vi "DCS_1_(Upgrade).vi"(3 "error in":errorcluster) -> (10 "error out":errorcluster)   [LabVIEW 2013]
uses:
  <vilib>/Utility/miscctls.llb/LVPointTypeDef.ctl
  <userlib>/Accelerator/User Interface/Controls/Role ID.ctl
  <userlib>/Accelerator/User Interface/Controls/dcs_spot.ctl
  <vilib>/gmath/NumericalOptimization/Nonlinear Curve Fit LM.vi
  <userlib>/Accelerator/User Interface/Controls/dcs points.ctl
  <vilib>/gmath/NI_Gmath.lvlib
panel:
  in  "Waveform Path":path=path "C:/Users/Chris/Desktop/DCS(Upgrade)/Waveforms"
  in  "Nornamiled":path=path "C:/Users/Chris/Desktop/DCS(Upgrade)/dcs_data/dcs_normalized.csv"
  in  "XY and Max":path=path "C:/Users/Chris/Desktop/DCS(Upgrade)/dcs_points/dcs_points.csv"
  in  "Points to Check Noise":i32=2000
  in  "Color bar Control":cluster{dbl, u32}[](array[cluster])
  in  "stop":bool
  in  "Tab Control":T1(tab)
  out "Intensity Graph":dbl[][](graph)
  in  "Spot Save Folder":path=path "C:/Users/Chris/Desktop/DCS(Upgrade)/dcs_data"
  in  "Save Spot Image":bool
  in  "Clear Spot/Track":bool
  in  "Particle Limit":i64=500 min=0 step=10
  out "Laser spot\nMove (mm)":dbl[](array[numeric])=[nan, nan] format="%#.3g"
  out "Avg. Freq. (Hz)":dbl
  in  "Orange Cursor Position":dbl[](array[numeric])=[0.0, 0.0] min=-12.0 max=12.0 step=0.1 format="%.3g"
  out "Spot Widths":dbl[](array[numeric]) format="%.6g"
  out "Countdown to\nnext track point":i32=1
  out "XY Graph":cluster{"Y":dbl[], "Y":dbl[]}[](graph)
  in  "Load old position\nto Orange Cursor":bool
  in  "Set Orange Cursor\nto current position":bool
  out "# of Particles\nin Spot":dbl
  out "Current Spot Pos":dbl[](array[numeric])=[nan, nan] format="%.3g"
  in  "# of shots to calculate spot":i32=20
  out "Spot Size over time":dbl[][](graph)
  out "Filtered Signals":dbl[][](graph)
  out "Unfiltered Signals":ext[][](graph)
  in  "Record Normalized":bool
  in  "Record XY":bool
  in  "External Trigger":bool
  in  "Auto Threshold":bool
  out "Sampling Frequency":u16(ring) items=["40 MHz", "20 MHz", "10 MHz", "5 MHz", "2.5 MHz", "1 MHz", "100 kHz", "10 kHz"]
  out "Length of Sample":dbl caption="s" format="%^#_3g"
  out "Memory Address Pointer":ext
  out "Post trigger Size":ext
  out "Pretrigger Size":ext
  out "Trigger Generation register":i32=23 format="%.0b"
  out "status register":i8=4 format="%08b"
  out "control register":i16=23 format="%015b"
  in  "Posttrigger size":i32
  in  "Acquisition Rate":u16(ring) items=["40 MHz", "20 MHz", "10 MHz", "5 MHz", "2.5 MHz", "1 MHz", "100 kHz", "10 kHz"]
  in  "Pretrigger size":i32=1000
  in  "Rising or falling?":bool
  out "Running Errors":errorcluster
  in  "Jorger TR slot":i32=3
  in  "Timeout (# of Cycles)":i32=100
  in  "Channels":i32[](array[numeric])=[0, 1, 2, 3, 4, 5, 6, 7]
  in  "Median Filter Rank":i32=30
  in  "Thresholds":ext[](array[numeric])
  in  "Level Buffer":i32=25
  # "DAQ Parameter Indicators"
  # "DAQ Parameter Controls"
  # "Falling"
  # "Rising"
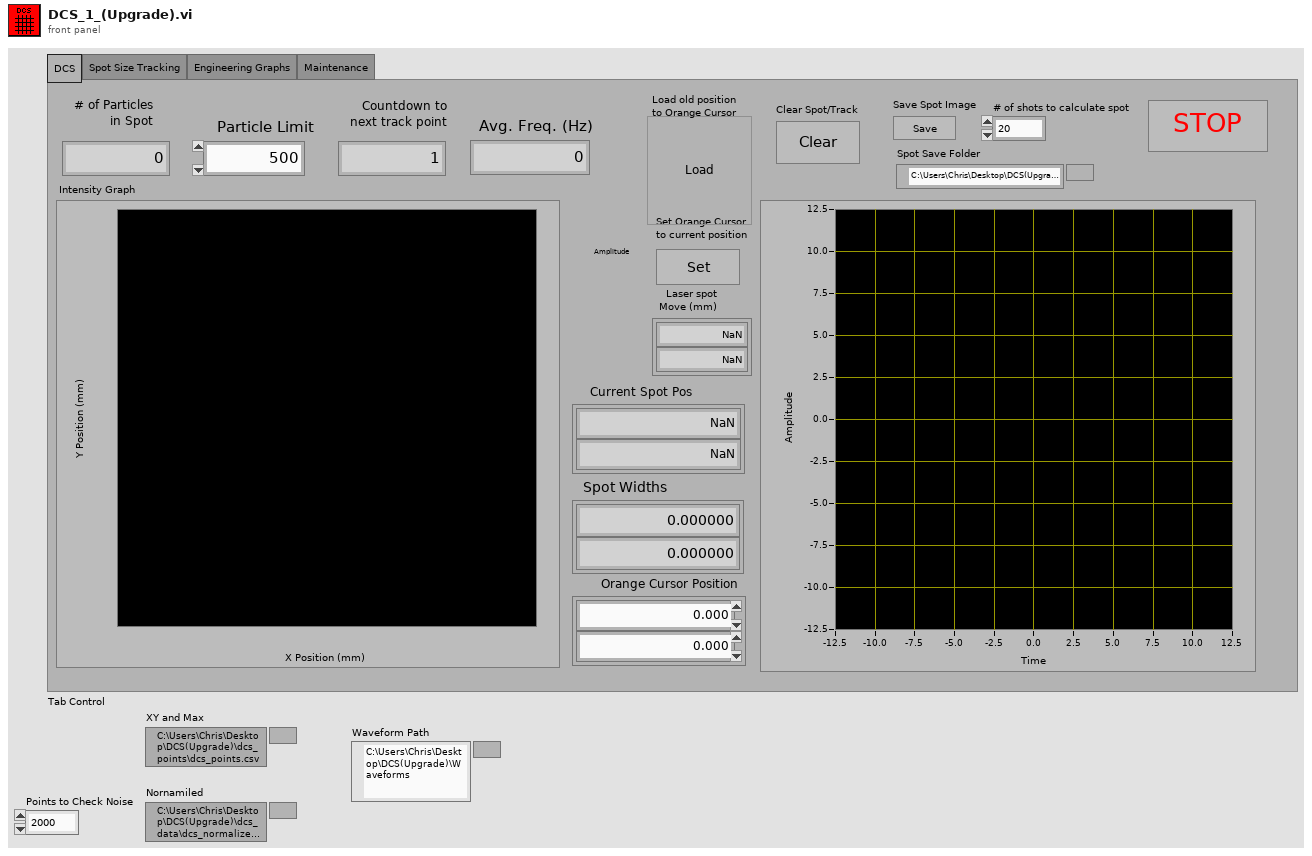
[diagram p1: front panel]
types:
  T1 = enum32{"DCS", "Spot Size Tracking", "Engineering Graphs", "Maintenance"}
  T2 = typedef "LVPointTypeDef.ctl" = cluster{"Horizontal":i16, "Vertical":i16}
  T3 = typedef "dcs_spot.ctl" = cluster{"DCS spot ID":i32, "Integer Timestamp":i64, "Spot X":dbl, "Spot Y":dbl, "Spot Width X":dbl, "Spot Width Y":dbl, "Spot Size":i32, "Experiment Settings ID":i32}
  T4 = typedef "Role ID.ctl" = enum16{"First_Detector", "Second_Detector", "Third_Detector", "LeCroy_CH1", "LeCroy_CH2", "LeCroy_CH3", "LeCroy_CH4", "PSU", "DCS 1", "DCS 2"}
  T5 = cluster{"Data":dbl[][], "Integer Timestamp":u64, "Signal Length":u32, "DCS_ID":u64, "Role ID":T4}
  T6 = typedef "dcs points.ctl" = cluster{"Integer Timestamp":i64, "X":dbl, "Y":dbl, "DCS spot ID":i32}
  T7 = cluster{"Data":dbl[][], "Integer Timestamp":u64, "Signal Length":u32, "DCS_ID":u64, "Role ID":T4}[]
  T8 = typedef "imagedata.ctl" = cluster{"image type":i32, "image depth":i32, "image":u8[], "mask":u8[], "colors":u32[], "Rectangle":cluster{"left":i16, "top":i16, "right":i16, "bottom":i16}}
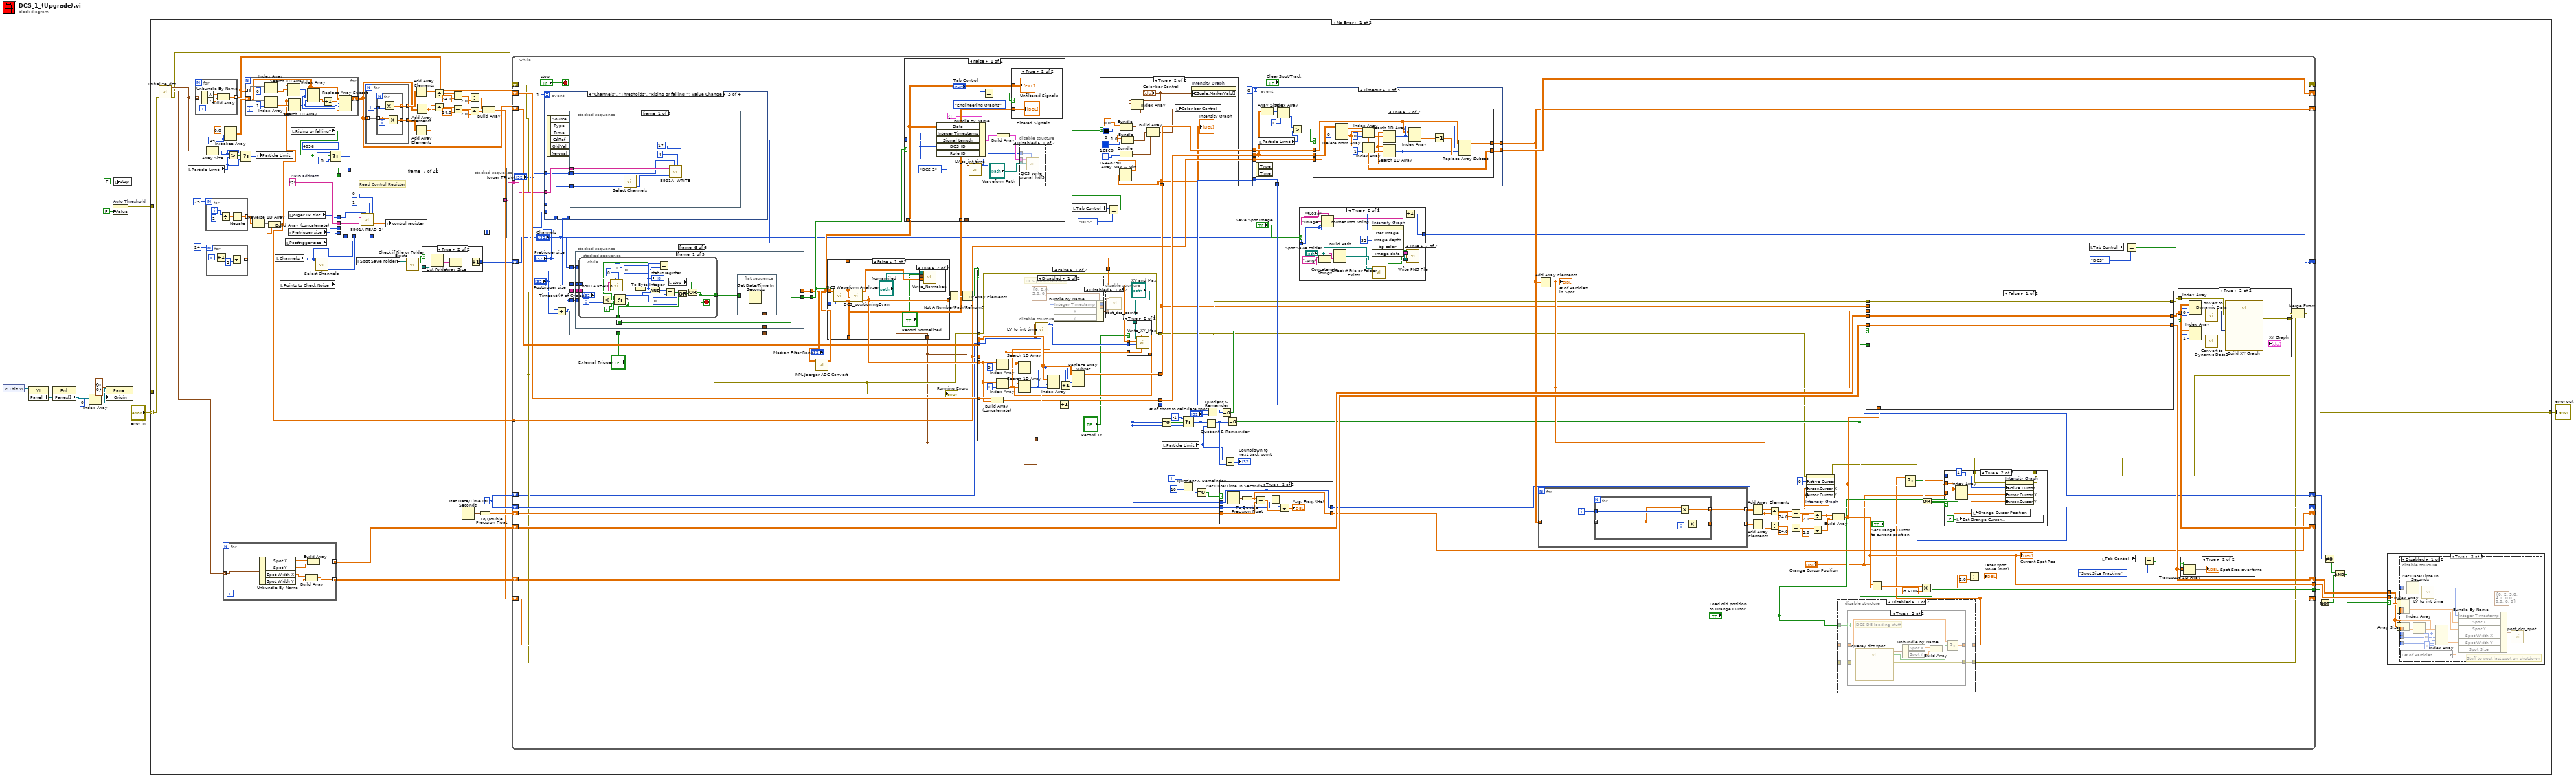
[diagram p0: block diagram]
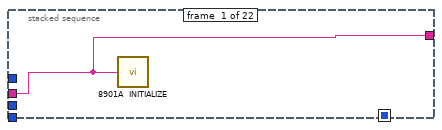
[diagram p2: hidden frame]
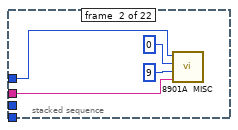
[diagram p3: hidden frame]
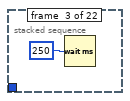
[diagram p4: hidden frame]
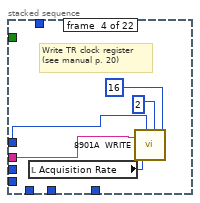
[diagram p5: hidden frame]
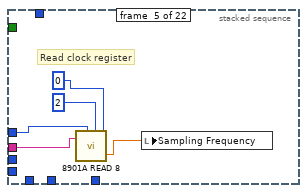
[diagram p6: hidden frame]
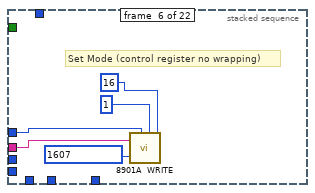
[diagram p7: hidden frame]
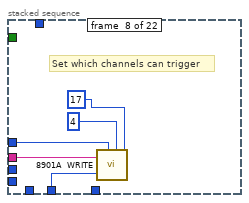
[diagram p8: hidden frame]
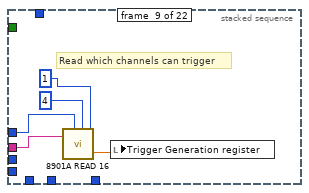
[diagram p9: hidden frame]
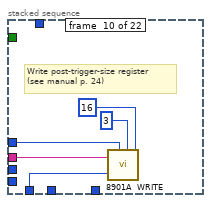
[diagram p10: hidden frame]
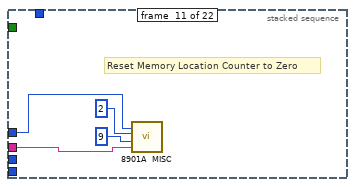
[diagram p11: hidden frame]
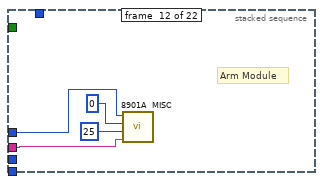
[diagram p12: hidden frame]
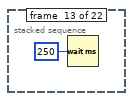
[diagram p13: hidden frame]
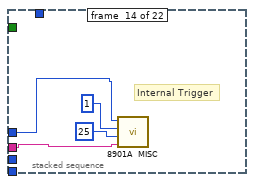
[diagram p14: hidden frame]
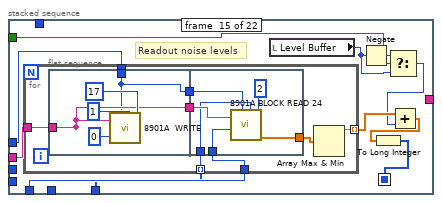
[diagram p15: hidden frame]
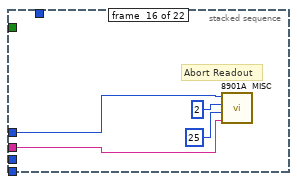
[diagram p16: hidden frame]
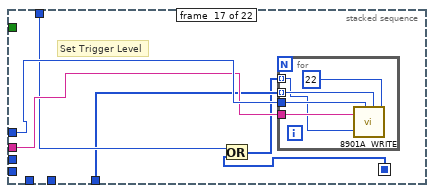
[diagram p17: hidden frame]
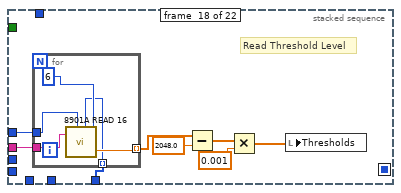
[diagram p18: hidden frame]
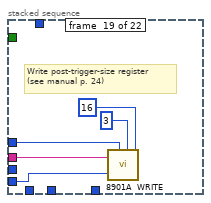
[diagram p19: hidden frame]
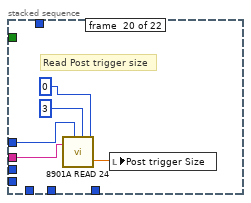
[diagram p20: hidden frame]
diagram:
  n1 = control-ref of="This VI"() -> (w11:refnum<vi>)
  n2 = property class="VI"(reference=w11) -> (error out=w10:errorcluster, "Panel"=w9:refnum<vi>)  [unwired: 1 in, 1 out]
  n3 = property class="Pnl"(reference=w9, error in=w10) -> (error out=w8:errorcluster, "Panes[]"=w7:refnum<vi>[])  [unwired: 1 out]
  n4 = Index Array(array=w7, index=0) -> (element=w5:refnum<vi>)
  n5 = property class="Pane"(reference=w5, error in=w8, "Origin"=T2 {"Horizontal"=0, "Vertical"=0}) -> (error out=w3:errorcluster)  [unwired: 1 out]
  n6 = property on="Auto Threshold" class="Bool (strict)"("Value"=FALSE ("Auto Threshold")) -> (error out=w1:errorcluster)  [unwired: 2 in, 1 out]
  n7 = local write "stop"(FALSE ("stop")) -> ()
  n8 = case shown="No Error" "error in" {
    selector: "error in" -> [w33 w976]
    tunnel: [w32 w976] -> w13
    tunnel: w3 -> [_ _]
    tunnel: w1 -> [_ _]
    frame No Error {
      w26 = "2"  # GPIB address
      w53 = 49 ("dimension size")
      w56 = 0
      n9 = call <userlib>:"initialize_dcs.vi"("error in (no error)"=w33) -> ("error out"=w27:errorcluster, "Dust Spot Array"=w45:T3[], "Dust Point Array"=w38:T6[])  [unwired: 8 in]
      n10 = local read "Particle Limit"() -> (w35:i64)
      n11 = for {
        tunnel: [w236] -> w44 mode=indexing
        tunnel: w38 -> [w235] mode=indexing
        n12 = Unbundle By Name(w235) -> ("X"=w238:dbl, "Y"=w237:dbl)
        n13 = Build Array(w238, w237) -> (w236:dbl[])
      }
      n14 = for {
        N: 25 -> [_]
        tunnel: [w274] -> w76 mode=indexing
        i -> [w277]
        n15 = Divide(x=w277, y=2) -> (x/y=w275:dbl)
        n16 = Negate(x=w275) -> (-x=w274:dbl)
      }
      n17 = Array Size(array=w38) -> (size(s)=w36:i32)
      n18 = for {
        N: 24 -> [_]
        tunnel: [w271] -> w74 mode=indexing
        i -> [w273]
        n19 = Increment(x=w273) -> (x+1=w270:i32)
        n20 = Divide(x=w270, y=2) -> (x/y=w271:dbl)
      }
      n21 = for {
        tunnel: [w230] -> w48 mode=indexing
        tunnel: [w229] -> w49 mode=indexing
        tunnel: w45 -> [w228] mode=indexing
        n22 = Unbundle By Name(w228) -> ("Spot X"=w234:dbl, "Spot Y"=w233:dbl, "Spot Width X"=w232:dbl, "Spot Width Y"=w231:dbl)
        n23 = Build Array(w232, w231) -> (w230:dbl[])
        n24 = Build Array(w234, w233) -> (w229:dbl[])
      }
      n25 = Initialize Array(0.0 ("element"), w53, w53) -> (w52:dbl[][])
      n26 = Greater?(x=w36, y=w35) -> (0:w37:bool)
      n27 = Select(t=w36, s=w37, f=w35) -> (s? t:f=w34:i64)
      n28 = Reverse 1D Array(array=w76) -> (reversed array=w75:dbl[])
      n29 = local write "Particle Limit"(w34) -> ()
      n30 = Build Array (concatenate)(w75, w74) -> (w50:dbl[])
      n31 = for {
        tunnel: w44 -> [w225] mode=indexing
        tunnel: w50 -> [w216]
        shift-right: [w217] -> w43
        shift-left: w52 -> [w218]
        n32 = Index Array(array=w225, index=0) -> (element=w224:dbl)
        n33 = Index Array(array=w225, index=1) -> (element=w223:dbl)
        n34 = Search 1D Array(1D array=w216, element=w224) -> (index of element=w220:i32)  [unwired: 1 in]
        n35 = Search 1D Array(1D array=w216, element=w223) -> (index of element=w219:i32)  [unwired: 1 in]
        n36 = Index Array(array=w218, index (row)=w220, index (col)=w219) -> (element=w222:dbl)
        n37 = Increment(x=w222) -> (x+1=w221:dbl)
        n38 = Replace Array Subset(array=w218, new element=w221, index (row)=w220, index (col)=w219) -> (w217:dbl[][])
      }
      n39 = local read "Channels"() -> (w17:i32[])
      n40 = local read "Points to Check Noise"() -> (w16:i32)
      n41 = local read "Posttrigger size"() -> (w22:i32)
      n42 = local read "Jorger TR slot"() -> (w24:i32)
      n43 = local read "Pretrigger size"() -> (w23:i32)
      n44 = local read "Rising or falling?"() -> (w15:bool)
      n45 = call <userlib>:"Select Channels.vi"("Channels"=w17) -> ("Channels in Use"=w21:u32)  [unwired: 10 in]
      n46 = Select(t=4096, s=w15, f=0) -> (s? t:f=w18:i32)
      n47 = stacked-sequence {
        seq-local: [_ _ _ _ _ _ _ _ _ _ _ _ _ _ w137 _ _ _ _ _ _ _] -> [_ _ _ _ _ _ _ _ _ _ _ _ _ _ _ _ w167 _ _ _ _ _]
        tunnel: w24 -> [_ w80 _ w87 w92 w95 w102 w106 w111 w117 w121 w124 _ w129 w139 w164 w172 w185 w193 w198 w203 w208]
        tunnel: w26 -> [w79 w81 _ w86 w91 w96 w101 w107 w112 w116 w120 w125 _ w130 w143 w163 w171 w184 w192 w197 w202 w207]
        tunnel: w23 -> [_ _ _ _ _ _ _ _ _ _ _ _ _ _ _ _ _ _ _ _ w201 _]
        tunnel: w22 -> [_ _ _ _ _ _ _ _ _ _ _ _ _ _ _ _ _ _ w191 _ _ _]
        tunnel: [w79 _ _ _ _ _ _ _ _ _ _ _ _ _ _ _ _ _ _ _ _ _] -> w25
        tunnel: w21 -> [_ _ _ _ _ _ _ w105 _ _ _ _ _ _ _ _ _ _ _ _ _ _]
        tunnel: w16 -> [_ _ _ _ _ _ _ _ _ w115 _ _ _ _ w142 _ _ _ _ _ _ _]
        tunnel: w18 -> [_ _ _ _ _ _ _ _ _ _ _ _ _ _ _ _ w170 _ _ _ _ _]
        tunnel: w17 -> [_ _ _ _ _ _ _ _ _ _ _ _ _ _ w140 _ w169 w179 _ _ _ _]
        tunnel: w15 -> [_ _ _ _ _ _ _ _ _ _ _ _ _ _ w134 _ _ _ _ _ _ _]
        frame #0 {
          n48 = call <instrlib>:"8901A  INITIALIZE.vi"("GPIB address"=w79) -> ()
        }
        frame #1 {
          n49 = call <instrlib>:"8901A  MISC.vi"("GPIB address"=w81, "f"=9, "a"=0, "n"=w80) -> ()
        }
        frame #2 {
          n50 = Wait (ms)(milliseconds to wait=250) -> ()  [unwired: 1 out]
        }
        frame #3 {
          # "Write TR clock register\n(see manual p. 20)"
          n51 = local read "Acquisition Rate"() -> (w85:u16)
          n52 = call <instrlib>:"8901A  WRITE.vi"("data"=w85, "GPIB address"=w86, "n"=w87, "a"=2, "f"=16) -> ()  [unwired: 1 in]
        }
        frame #4 {
          # "Read clock register"
          n53 = call <instrlib>:"8901A READ 8.vi"("GPIB address"=w91, "n"=w92, "a"=2, "f"=0) -> ("output"=w90:ext)  [unwired: 3 in]
          n54 = local write "Sampling Frequency"(w90) -> ()
        }
        frame #5 {
          # "Set Mode (control register no wrapping)"
          n55 = call <instrlib>:"8901A  WRITE.vi"("data"=1607, "GPIB address"=w96, "n"=w95, "a"=1, "f"=16) -> ()  [unwired: 1 in]
        }
        frame #6 {
          # "Read Control Register"
          n56 = call <instrlib>:"8901A READ 24.vi"("GPIB address"=w101, "n"=w102, "a"=1, "f"=0) -> ("output"=w100:ext)  [unwired: 3 in]
          n57 = local write "control register"(w100) -> ()
        }
        frame #7 {
          # "Set which channels can trigger"
          n58 = call <instrlib>:"8901A  WRITE.vi"("data"=w105, "GPIB address"=w107, "n"=w106, "a"=4, "f"=17) -> ()  [unwired: 1 in]
        }
        frame #8 {
          # "Read which channels can trigger"
          n59 = call <instrlib>:"8901A READ 16.vi"("GPIB address"=w112, "n"=w111, "a"=u8 4, "f"=u8 1) -> ("output"=w110:ext)  [unwired: 3 in]
          n60 = local write "Trigger Generation register"(w110) -> ()
        }
        frame #9 {
          # "Write post-trigger-size register\n(see manual p. 24)"
          n61 = call <instrlib>:"8901A  WRITE.vi"("data"=w115, "GPIB address"=w116, "n"=w117, "a"=3, "f"=16) -> ()  [unwired: 1 in]
        }
        frame #10 {
          # "Reset Memory Location Counter to Zero"
          n62 = call <instrlib>:"8901A  MISC.vi"("GPIB address"=w120, "f"=u8 9, "a"=u8 2, "n"=w121) -> ()
        }
        frame #11 {
          # "Arm Module"
          n63 = call <instrlib>:"8901A  MISC.vi"("GPIB address"=w125, "f"=25, "a"=0, "n"=w124) -> ()
        }
        frame #12 {
          n64 = Wait (ms)(milliseconds to wait=u32 250) -> ()  [unwired: 1 out]
        }
        frame #13 {
          # "Internal Trigger"
          n65 = call <instrlib>:"8901A  MISC.vi"("GPIB address"=w130, "f"=u8 25, "a"=u8 1, "n"=w129) -> ()
        }
        frame #14 {
          # "Readout noise levels"
          n66 = for {
            tunnel: w143 -> [w150]
            tunnel: w142 -> [w149]
            tunnel: [w147] -> w141 mode=indexing
            tunnel: w140 -> [w146] mode=indexing
            tunnel: w139 -> [w145]
            n67 = flat-sequence {
              tunnel: [w154] -> _
              tunnel: [w154] -> w151
              tunnel: w150 -> [w154]
              tunnel: w145 -> [w152]
              tunnel: [w152] -> w144
              tunnel: w151 -> [w161]
              tunnel: [w160] -> w148
              tunnel: w149 -> [w159]
              tunnel: w146 -> [w158]
              tunnel: w144 -> [w157]
              frame #0 {
                n68 = call <instrlib>:"8901A  WRITE.vi"("data"=0, "GPIB address"=w154, "n"=w152, "a"=1, "f"=17) -> ()  [unwired: 1 in]
              }
              frame #1 {
                n69 = call <instrlib>:"8901A BLOCK READ 24.vi"("f"=2, "a"=w158, "n"=w157, "GPIB address"=w161, "# points to read"=w159) -> ("output"=w160:ext[])  [unwired: 4 in]
              }
            }
            n70 = Array Max & Min(array=w148) -> (max value=w147:ext)  [unwired: 3 out]
          }
          n71 = local read "Level Buffer"() -> (w136:i32)
          n72 = Negate(x=w136) -> (-x=w135:i32)
          n73 = Select(t=w135, s=w134, f=w136) -> (s? t:f=w133:i32)
          n74 = Add(x=w141, y=w133) -> (x+y=w138:ext[])
          n75 = To Long Integer(number=w138) -> (32bit integer=w137:i32[])
        }
        frame #15 {
          # "Abort Readout"
          n76 = call <instrlib>:"8901A  MISC.vi"("GPIB address"=w163, "f"=25, "a"=2, "n"=w164) -> ()
        }
        frame #16 {
          # "Set Trigger Level"
          n77 = Or(x=w170, y=w167) -> (x .or. y?=w168:i32[])
          n78 = for {
            tunnel: w172 -> [w176]
            tunnel: w171 -> [w175]
            tunnel: w169 -> [w174] mode=indexing
            tunnel: w168 -> [w173] mode=indexing
            n79 = call <instrlib>:"8901A  WRITE.vi"("data"=w173, "GPIB address"=w175, "n"=w176, "a"=w174, "f"=u8 22) -> ()  [unwired: 1 in]
          }
        }
        frame #17 {
          # "Read Threshold Level"
          n80 = for {
            tunnel: w185 -> [w189]
            tunnel: w184 -> [w188]
            tunnel: [w187] -> w182 mode=indexing
            tunnel: w179 -> [w186] mode=indexing
            n81 = call <instrlib>:"8901A READ 16.vi"("GPIB address"=w188, "n"=w189, "a"=w186, "f"=u8 6) -> ("output"=w187:ext)  [unwired: 3 in]
          }
          n82 = Subtract(x=w182, y=2048.0) -> (x-y=w180:ext[])
          n83 = Multiply(x=w180, y=0.001) -> (x*y=w178:ext[])
          n84 = local write "Thresholds"(w178) -> ()
        }
        frame #18 {
          # "Write post-trigger-size register\n(see manual p. 24)"
          n85 = call <instrlib>:"8901A  WRITE.vi"("data"=w191, "GPIB address"=w192, "n"=w193, "a"=3, "f"=16) -> ()  [unwired: 1 in]
        }
        frame #19 {
          # "Read Post trigger size"
          n86 = call <instrlib>:"8901A READ 24.vi"("GPIB address"=w197, "n"=w198, "a"=3, "f"=0) -> ("output"=w196:ext)  [unwired: 3 in]
          n87 = local write "Post trigger Size"(w196) -> ()
        }
        frame #20 {
          # "Write Pretrigger size"
          n88 = call <instrlib>:"8901A  WRITE.vi"("data"=w201, "GPIB address"=w202, "n"=w203, "a"=4, "f"=16) -> ()  [unwired: 1 in]
        }
        frame #21 {
          # "Read Pretrigger size"
          n89 = call <instrlib>:"8901A READ 16.vi"("GPIB address"=w207, "n"=w208, "a"=u8 4, "f"=u8 0) -> ("output"=w206:ext)  [unwired: 3 in]
          n90 = local write "Pretrigger Size"(w206) -> ()
        }
      }
      n91 = local read "Spot Save Folder"() -> (w30:path)
      n92 = for {
        tunnel: w43 -> [w264] mode=indexing
        tunnel: [w262] -> w73 mode=indexing
        tunnel: [w261] -> w72 mode=indexing
        i -> [w263]
        n93 = for {
          tunnel: w264 -> [w266] mode=indexing
          tunnel: w263 -> [w269]
          tunnel: [w267] -> w261 mode=indexing
          tunnel: [w265] -> w262 mode=indexing
          i -> [w268]
          n94 = Multiply(x=w266, y=w269) -> (x*y=w265:dbl)
          n95 = Multiply(x=w266, y=w268) -> (x*y=w267:dbl)
        }
      }
      n96 = call <vilib>:"Check if File or Folder Exists.vi"("path"=w30) -> ("file or folder exists?"=w29:bool, "dup path"=w28:path)  [unwired: 8 in, 1 out]
      n97 = Add Array Elements(numeric array=w73) -> (sum=w71:dbl)
      n98 = Add Array Elements(numeric array=w72) -> (sum=w70:dbl)
      n99 = Add Array Elements(numeric array=w43) -> (sum=w62:dbl)
      n100 = case shown="True" w29 {
        tunnel: [0 w213] -> w31
        tunnel: w28 -> [_ w212]
        frame False {
        }
        frame True {
          n101 = List Folder(path=w212) -> (filenames=w215:string[])  [unwired: 3 in, 3 out]
          n102 = Array Size(array=w215) -> (size(s)=w214:i32)
          n103 = Increment(x=w214) -> (x+1=w213:i32)
        }
      }
      n104 = Divide(x=w71, y=w62) -> (x/y=w69:dbl)
      n105 = Divide(x=w70, y=w62) -> (x/y=w68:dbl)
      n106 = Subtract(x=w69, y=24.0) -> (x-y=w60:dbl)
      n107 = Subtract(x=w68, y=24.0) -> (x-y=w66:dbl)
      n108 = Get Date/Time In Seconds() -> (seconds since 1Jan1904=w58:timestamp)
      n109 = Divide(x=w60, y=2.0) -> (x/y=w59:dbl)
      n110 = Divide(x=w66, y=2.0) -> (x/y=w63:dbl)
      n111 = To Double Precision Float(number=w58) -> (double precision float=w57:dbl)
      n112 = Build Array(w59, w63) -> (w51:dbl[])
      n113 = while {
        shift-right: [w356] -> _
        shift-left: w44 -> [w358]
        shift-right: [w341] -> _
        shift-left: w43 -> [w380]
        tunnel: w50 -> [w332]
        shift-right: [w340] -> _
        shift-left: w51 -> [w368]
        tunnel: [w355] -> w55
        shift-right: [w331] -> w32
        shift-left: w27 -> [w293]
        shift-right: [w353] -> _
        shift-left: w49 -> [w345]
        shift-right: [w325] -> w42
        shift-left: w56 -> [w280]
        shift-right: [w354] -> w46
        shift-left: w48 -> [w357]
        shift-right: [w338] -> _
        shift-left: w57 -> [w352]
        shift-right: [w337] -> _
        shift-left: w56 -> [w339]
        tunnel: [w322] -> w47
        shift-right: [w282] -> _
        shift-left: w31 -> [w281]
        tunnel: w25 -> [w297]
        i -> [w308]
        stop <- "stop" stop-if-true
        n114 = event shown="[2] \"Channels\", \"Thresholds\", \"Rising or falling?\": Value Change" {
          selector: _ -> [_ _ _ _]
          dyn-events: _ -> [_ _ _ _]
          timeout: 1 -> [_ _ _ _]
          tunnel: w297 -> [_ w551 w616 w652]
          tunnel: "Pretrigger size" -> [_ w550 _ _]
          tunnel: "Posttrigger size" -> [_ w549 _ w647]
          tunnel: [w538 w539 w615 w649] -> w296
          tunnel: "Channels" -> [_ w541 w614 w650]
          tunnel: "Jorger TR slot" -> [_ w539 w615 w649]
          event Timeout {
            n115 = event-data() -> ()  [unwired: 1 in, 3 out]
            n116 = local read "Jorger TR slot"() -> (w538:i32)
          }
          event "Acquisition Rate", "Pretrigger size", "Posttrigger size": Value Change {
            n117 = event-data() -> ()  [unwired: 1 in, 6 out]
            n118 = local read "Acquisition Rate"() -> (w548:u16)
            n119 = call <userlib>:"Select Channels.vi"("Channels"=w541) -> ("Channels in Use"=w540:u32)  [unwired: 10 in]
            n120 = stacked-sequence {
              tunnel: w539 -> [w586 w591 w596 w601 w606 w611]
              tunnel: w551 -> [w585 w590 w595 w600 w605 w610]
              tunnel: w550 -> [_ _ _ _ w604 _]
              tunnel: w549 -> [w584 _ _ _ _ _]
              tunnel: w540 -> [_ _ _ _ _ _]
              frame #0 {
                # "Write post-trigger-size register\n(see manual p. 24)"
                n121 = call <instrlib>:"8901A  WRITE.vi"("data"=w584, "GPIB address"=w585, "n"=w586, "a"=3, "f"=16) -> ()  [unwired: 1 in]
              }
              frame #1 {
                # "Read Post trigger size"
                n122 = call <instrlib>:"8901A READ 24.vi"("GPIB address"=w590, "n"=w591, "a"=3, "f"=0) -> ("output"=→"Post trigger Size":ext)  [unwired: 3 in]
              }
              frame #2 {
                # "Write TR clock register\n(see manual p. 20)"
                n123 = call <instrlib>:"8901A  WRITE.vi"("data"="Acquisition Rate", "GPIB address"=w595, "n"=w596, "a"=2, "f"=16) -> ()  [unwired: 1 in]
              }
              frame #3 {
                # "Read clock register"
                n124 = call <instrlib>:"8901A READ 8.vi"("GPIB address"=w600, "n"=w601, "a"=2, "f"=0) -> ("output"=→"Sampling Frequency":ext)  [unwired: 3 in]
              }
              frame #4 {
                # "Write Pretrigger size"
                n125 = call <instrlib>:"8901A  WRITE.vi"("data"=w604, "GPIB address"=w605, "n"=w606, "a"=4, "f"=16) -> ()  [unwired: 1 in]
              }
              frame #5 {
                # "Read Pretrigger size"
                n126 = call <instrlib>:"8901A READ 16.vi"("GPIB address"=w610, "n"=w611, "a"=u8 4, "f"=u8 0) -> ("output"=→"Pretrigger Size":ext)  [unwired: 3 in]
              }
            }
            n127 = case shown="0, Default" w548 {
              tunnel: [w552 w556 w560 w564 w568 w572 w576 w580] -> w546
              frame 0, Default {
                n128 = Power Of 10(x=6) -> (10^x=w554:dbl)
                n129 = Multiply(x=40, y=w554) -> (x*y=w552:dbl)
              }
              frame 1 {
                n130 = Power Of 10(x=6) -> (10^x=w558:dbl)
                n131 = Multiply(x=20, y=w558) -> (x*y=w556:dbl)
              }
              frame 2 {
                n132 = Power Of 10(x=6) -> (10^x=w562:dbl)
                n133 = Multiply(x=10, y=w562) -> (x*y=w560:dbl)
              }
              frame 3 {
                n134 = Power Of 10(x=6) -> (10^x=w566:dbl)
                n135 = Multiply(x=5, y=w566) -> (x*y=w564:dbl)
              }
              frame 4 {
                n136 = Power Of 10(x=6) -> (10^x=w570:dbl)
                n137 = Multiply(x=2.5, y=w570) -> (x*y=w568:dbl)
              }
              frame 5 {
                n138 = Power Of 10(x=6) -> (10^x=w574:dbl)
                n139 = Multiply(x=1, y=w574) -> (x*y=w572:dbl)
              }
              frame 6 {
                n140 = Power Of 10(x=3) -> (10^x=w578:dbl)
                n141 = Multiply(x=100, y=w578) -> (x*y=w576:dbl)
              }
              frame 7 {
                n142 = Power Of 10(x=3) -> (10^x=w582:dbl)
                n143 = Multiply(x=10, y=w582) -> (x*y=w580:dbl)
              }
            }
            n144 = local read "Posttrigger size"() -> (w545:i32)
            n145 = Reciprocal(x=w546) -> (1/x=w547:dbl)
            n146 = local read "Pretrigger size"() -> (w544:i32)
            n147 = Add(x=w545, y=w544) -> (x+y=w543:i32)
            n148 = Multiply(x=w543, y=w547) -> (x*y=→"Length of Sample":dbl)
          }
          event "Channels", "Thresholds", "Rising or falling?": Value Change {
            n149 = event-data() -> ()  [unwired: 1 in, 6 out]
            n150 = stacked-sequence {
              tunnel: w616 -> [w620 w624 w632]
              tunnel: w615 -> [w619 w625 w631]
              tunnel: w614 -> [w617 _ w630]
              frame #0 {
                n151 = call <userlib>:"Select Channels.vi"("Channels"=w617) -> ("Channels in Use"=w618:u32)  [unwired: 10 in]
                n152 = call <instrlib>:"8901A  WRITE.vi"("data"=w618, "GPIB address"=w620, "n"=w619, "a"=4, "f"=17) -> ()  [unwired: 1 in]
              }
              frame #1 {
                n153 = call <instrlib>:"8901A READ 16.vi"("GPIB address"=w624, "n"=w625, "a"=u8 4, "f"=u8 1) -> ("output"=→"Trigger Generation register":ext)  [unwired: 3 in]
              }
              frame #2 {
                n154 = Add(x="Thresholds", y=2.048) -> (x+y=w640:ext[])
                n155 = Multiply(x=w640, y=1000.0) -> (x*y=w638:ext[])
                n156 = Select(t=4096, s="Rising or falling?", f=0) -> (s? t:f=w634:i32)
                n157 = To Long Integer(number=w638) -> (32bit integer=w635:i32[])
                n158 = Or(x=w634, y=w635) -> (x .or. y?=w633:i32[])
                n159 = for {
                  tunnel: w631 -> [w645]
                  tunnel: w632 -> [w644]
                  tunnel: w630 -> [w643] mode=indexing
                  tunnel: w633 -> [w642] mode=indexing
                  n160 = call <instrlib>:"8901A  WRITE.vi"("data"=w642, "GPIB address"=w644, "n"=w645, "a"=w643, "f"=u8 22) -> ()  [unwired: 1 in]
                }
              }
            }
          }
          event "Auto Threshold": Value Change {
            n161 = event-data() -> ()  [unwired: 1 in, 6 out]
            n162 = stacked-sequence {
              seq-local: [_ _ _ _ _ _ _ w682 _ _ _ _] -> [_ _ _ _ _ _ _ _ _ w715 _ _]
              tunnel: w652 -> [w655 w659 w663 w667 w671 _ w676 w686 w710 w717 w730 w743]
              tunnel: "Points to Check Noise" -> [w654 _ _ _ _ _ _ w684 _ _ _ _]
              tunnel: w649 -> [w653 w658 w664 w668 w672 _ w677 w685 w711 w716 w729 w742]
              tunnel: w650 -> [_ _ _ _ _ _ _ w683 _ w718 w731 _]
              tunnel: w647 -> [_ _ _ _ _ _ _ _ _ _ _ w741]
              frame #0 {
                # "Write post-trigger-size register\n(see manual p. 24)"
                n163 = call <instrlib>:"8901A  WRITE.vi"("data"=w654, "GPIB address"=w655, "n"=w653, "a"=3, "f"=16) -> ()  [unwired: 1 in]
              }
              frame #1 {
                # "Turn off Wrapping"
                n164 = call <instrlib>:"8901A  WRITE.vi"("data"=1607, "GPIB address"=w659, "n"=w658, "a"=1, "f"=16) -> ()  [unwired: 1 in]
              }
              frame #2 {
                # "Reset Memory Counter to Zero"
                n165 = call <instrlib>:"8901A  MISC.vi"("GPIB address"=w663, "f"=u8 9, "a"=u8 2, "n"=w664) -> ()
              }
              frame #3 {
                # "Arm Module"
                n166 = call <instrlib>:"8901A  MISC.vi"("GPIB address"=w667, "f"=25, "a"=0, "n"=w668) -> ()
              }
              frame #4 {
                n167 = call <instrlib>:"8901A  MISC.vi"("GPIB address"=w671, "f"=u8 21, "a"=u8 2, "n"=w672) -> ()
              }
              frame #5 {
                n168 = Wait (ms)(milliseconds to wait=u32 250) -> ()  [unwired: 1 out]
              }
              frame #6 {
                # "Internal Trigger"
                n169 = call <instrlib>:"8901A  MISC.vi"("GPIB address"=w676, "f"=u8 25, "a"=u8 1, "n"=w677) -> ()
              }
              frame #7 {
                n170 = for {
                  tunnel: w686 -> [w697]
                  tunnel: w684 -> [w696]
                  tunnel: [w694] -> w690 mode=indexing
                  tunnel: w683 -> [w693] mode=indexing
                  tunnel: w685 -> [w692]
                  n171 = flat-sequence {
                    tunnel: [w701] -> _
                    tunnel: [w701] -> w698
                    tunnel: w697 -> [w701]
                    tunnel: w692 -> [w699]
                    tunnel: [w699] -> w691
                    tunnel: w698 -> [w708]
                    tunnel: [w707] -> w695
                    tunnel: w696 -> [w706]
                    tunnel: w693 -> [w705]
                    tunnel: w691 -> [w704]
                    frame #0 {
                      n172 = call <instrlib>:"8901A  WRITE.vi"("data"=0, "GPIB address"=w701, "n"=w699, "a"=1, "f"=17) -> ()  [unwired: 1 in]
                    }
                    frame #1 {
                      n173 = call <instrlib>:"8901A BLOCK READ 24.vi"("f"=2, "a"=w705, "n"=w704, "GPIB address"=w708, "# points to read"=w706) -> ("output"=w707:ext[])  [unwired: 4 in]
                    }
                  }
                  n174 = Array Max & Min(array=w695) -> (max value=w694:ext)  [unwired: 3 out]
                }
                n175 = local read "Rising or falling?"() -> (w680:bool)
                n176 = Negate(x="Level Buffer") -> (-x=w688:i32)
                n177 = Select(t=w688, s=w680, f="Level Buffer") -> (s? t:f=w687:i32)
                n178 = Add(x=w690, y=w687) -> (x+y=w689:ext[])
                n179 = To Long Integer(number=w689) -> (32bit integer=w682:i32[])
              }
              frame #8 {
                # "Abort Readout"
                n180 = call <instrlib>:"8901A  MISC.vi"("GPIB address"=w710, "f"=25, "a"=2, "n"=w711) -> ()
              }
              frame #9 {
                n181 = local read "Rising or falling?"() -> (w714:bool)
                n182 = Select(t=4096, s=w714, f=0) -> (s? t:f=w719:i32)
                n183 = Or(x=w719, y=w715) -> (x .or. y?=w722:i32[])
                n184 = for {
                  tunnel: w716 -> [w726]
                  tunnel: w717 -> [w725]
                  tunnel: w718 -> [w724] mode=indexing
                  tunnel: w722 -> [w723] mode=indexing
                  n185 = call <instrlib>:"8901A  WRITE.vi"("data"=w723, "GPIB address"=w725, "n"=w726, "a"=w724, "f"=u8 22) -> ()  [unwired: 1 in]
                }
              }
              frame #10 {
                n186 = for {
                  tunnel: w729 -> [w739]
                  tunnel: w730 -> [w738]
                  tunnel: [w737] -> w732 mode=indexing
                  tunnel: w731 -> [w736] mode=indexing
                  n187 = call <instrlib>:"8901A READ 16.vi"("GPIB address"=w738, "n"=w739, "a"=w736, "f"=u8 6) -> ("output"=w737:ext)  [unwired: 3 in]
                }
                n188 = Subtract(x=w732, y=2048.0) -> (x-y=w733:ext[])
                n189 = Multiply(x=w733, y=0.001) -> (x*y=w728:ext[])
                n190 = local write "Thresholds"(w728) -> ()
              }
              frame #11 {
                # "Write post-trigger-size register\n(see manual p. 24)"
                n191 = call <instrlib>:"8901A  WRITE.vi"("data"=w741, "GPIB address"=w743, "n"=w742, "a"=3, "f"=16) -> ()  [unwired: 1 in]
              }
            }
            n192 = local write "Auto Threshold"(FALSE ("Auto Threshold")) -> ()
          }
        }
        n193 = Add(x="Pretrigger size", y="Posttrigger size") -> (x+y=w279:i32)
        n194 = stacked-sequence {
          tunnel: w296 -> [w432 w439 w443 w446 w450 w459]
          tunnel: w297 -> [w431 w438 w442 w447 w451 w460]
          tunnel: [_ _ _ _ _ w458] -> w290
          tunnel: w279 -> [_ _ _ _ _ w457]
          tunnel: "Channels" -> [_ _ _ _ _ w456]
          tunnel: [_ _ _ _ _ w455] -> w287
          tunnel: "External Trigger" -> [w429 _ _ _ _ _]
          tunnel: [_ _ _ _ _ w454] -> w278
          frame #0 {
            # "Set Control Register"
            n195 = case shown="True" w429 {
              tunnel: [1615 79 ("data")] -> w430
              frame False {
              }
              frame True {
              }
            }
            n196 = call <instrlib>:"8901A  WRITE.vi"("data"=w430, "GPIB address"=w431, "n"=w432, "a"=1, "f"=16) -> ()  [unwired: 1 in]
          }
          frame #1 {
            # "Read Control Register"
            n197 = call <instrlib>:"8901A READ 24.vi"("GPIB address"=w438, "n"=w439, "a"=1, "f"=0) -> ("output"=→"control register":ext)  [unwired: 3 in]
          }
          frame #2 {
            # "Reset Memory Location counter to 0"
            n198 = call <instrlib>:"8901A  MISC.vi"("GPIB address"=w442, "f"=u8 9, "a"=u8 2, "n"=w443) -> ()
          }
          frame #3 {
            # "Arm Module"
            n199 = call <instrlib>:"8901A  MISC.vi"("GPIB address"=w447, "f"=25, "a"=0, "n"=w446) -> ()
          }
          frame #4 {
            # "Clear All Valid Trigger tags"
            n200 = call <instrlib>:"8901A  MISC.vi"("GPIB address"=w451, "f"=u8 21, "a"=u8 2, "n"=w450) -> ()
          }
          frame #5 {
            n201 = stacked-sequence {
              seq-local: [w463 _ _ _ _] -> [_ w489 w500 _ _]
              tunnel: w460 -> [w465 w487 w497 w529 w534]
              tunnel: w459 -> [w464 w488 w496 w530 w535]
              tunnel: [w463 _ _ _ _] -> w458
              tunnel: w457 -> [_ _ w499 _ _]
              tunnel: w456 -> [_ _ w498 _ _]
              tunnel: [_ _ w495 _ _] -> w455
              tunnel: [w461 _ _ _ _] -> w454
              frame #0 {
                n202 = while {
                  tunnel: w465 -> [w479]
                  tunnel: w464 -> [w478]
                  tunnel: [w468] -> w463
                  tunnel: [w467] -> w462
                  i -> [w477]
                  stop <- w467 stop-if-true
                  n203 = Less?(x="Timeout (# of Cycles)", y=w477) -> (x < y?=w470:bool)
                  n204 = call <instrlib>:"8901A READ 8.vi"("GPIB address"=w479, "n"=w478, "a"=0, "f"=1) -> ("output"=w482:ext)  [unwired: 3 in]
                  n205 = To Byte Integer(number=w482) -> (8bit integer=w473:i8)
                  "status register" <- w473
                  n206 = And(x=w473, y=i8 3) -> (x .and. y?=w483:i8)
                  n207 = Equal?(x=w473, y=i8 0) -> (x = y?=w471:bool)
                  n208 = Select(t=TRUE, s=w471, f=w470) -> (s? t:f=w468:bool)
                  n209 = Equal?(x=w483, y=i8 0) -> (x = y?=w475:bool)
                  n210 = local read "stop"() -> (w474:bool)
                  n211 = Or(x=w475, y=w468) -> (x .or. y?=w484:bool)
                  n212 = Or(x=w474, y=w484) -> (x .or. y?=w467:bool)
                }
                n213 = flat-sequence {
                  tunnel: w462 -> [_]
                  tunnel: [w466] -> w461
                  frame #0 {
                    n214 = Get Date/Time In Seconds() -> (seconds since 1Jan1904=w466:timestamp)
                  }
                }
              }
              frame #1 {
                n215 = case shown="False" w489 {
                  tunnel: w488 -> [w492 _]
                  tunnel: w487 -> [w491 _]
                  frame False {
                    n216 = call <instrlib>:"8901A READ 24.vi"("GPIB address"=w491, "n"=w492, "a"=u8 9, "f"=u8 0) -> ("output"=→"Memory Address Pointer":ext)  [unwired: 3 in]
                  }
                  frame True {
                  }
                }
              }
              frame #2 {
                n217 = case shown="False" w500 {
                  tunnel: w499 -> [w505 _]
                  tunnel: w498 -> [w506 _]
                  tunnel: w497 -> [w504 _]
                  tunnel: w496 -> [w503 _]
                  tunnel: [w501 ext[][] [[nan]] ("output")] -> w495
                  frame False {
                    n218 = local read "Memory Address Pointer"() -> (w502:ext)
                    n219 = for {
                      N: 8 -> [_]
                      tunnel: w506 -> [w510] mode=indexing
                      tunnel: w505 -> [w509]
                      tunnel: w504 -> [w514]
                      tunnel: w503 -> [w513]
                      tunnel: w502 -> [w516]
                      tunnel: [w508] -> w501 mode=indexing
                      n220 = Subtract(x=w516, y=w509) -> (x-y=w515:ext)
                      n221 = flat-sequence {
                        tunnel: w515 -> [w519]
                        tunnel: w514 -> [w517]
                        tunnel: w513 -> [w518]
                        tunnel: [w518] -> w512
                        tunnel: [w517] -> w511
                        tunnel: w512 -> [w525]
                        tunnel: w511 -> [w524]
                        tunnel: w510 -> [w526]
                        tunnel: w509 -> [w523]
                        tunnel: [w522] -> w508
                        frame #0 {
                          n222 = call <instrlib>:"8901A  WRITE.vi"("data"=w519, "GPIB address"=w517, "n"=w518, "a"=1, "f"=17) -> ()  [unwired: 1 in]
                        }
                        frame #1 {
                          n223 = call <instrlib>:"8901A BLOCK READ 24.vi"("f"=2, "a"=w526, "n"=w525, "GPIB address"=w524, "# points to read"=w523) -> ("output"=w522:ext[])  [unwired: 4 in]
                        }
                      }
                    }
                  }
                  frame True {
                  }
                }
              }
              frame #3 {
                # "Abort Readout"
                n224 = call <instrlib>:"8901A  MISC.vi"("GPIB address"=w529, "f"=25, "a"=2, "n"=w530) -> ()
              }
              frame #4 {
                # "Read in control register"
                n225 = call <instrlib>:"8901A READ 24.vi"("GPIB address"=w534, "n"=w535, "a"=1, "f"=0) -> ("output"=w533:ext)  [unwired: 3 in]
                n226 = local write "control register"(w533) -> ()
              }
            }
          }
        }
        n227 = call <userlib>:"NPL Joerger ADC Convert.vi"("Input"=w287) -> ("Output"=w286:ext[][])  [unwired: 10 in]
        n228 = case shown="False" w290 {
          tunnel: [w423 w427] -> w365
          tunnel: w286 -> [w422 _]
          tunnel: "Median Filter Rank" -> [w421 _]
          tunnel: [w420 dbl[][] [] ("Filtered Signals")] -> w291
          tunnel: [w419 w427] -> w284
          tunnel: w278 -> [w416 _]
          frame False {
            n229 = call <userlib>:"DCS Waveform Analyzer.vi"("Rank"=w421, "8 DCS Waveforms"=w422) -> ("Filtered Signals"=w420:dbl[][], "Maxs"=w419:dbl[])  [unwired: 8 in]
            n230 = call <userlib>:"DCS_positioningEvan.vi"("Data"=w419) -> ("X-Y position"=w423:dbl[], "Normalized Data"=w417:dbl[][])  [unwired: 9 in]
            n231 = case shown="True" "Record Normalized" {
              tunnel: "Nornamiled" -> [_ w426]
              tunnel: w417 -> [_ w425]
              tunnel: w416 -> [_ w424]
              frame False {
              }
              frame True {
                n232 = call <userlib>:"Write_Normalize.vi"("Normalized Data"=w425, "seconds since 1Jan1904"=w424, "Nornamiled"=w426) -> ()  [unwired: 9 in]
              }
            }
          }
          frame True {
            w427 = dbl[] [nan] ("X-Y position")
          }
        }
        n233 = case shown="False" w290 {
          tunnel: w286 -> [w404 _]
          tunnel: w291 -> [w409 _]
          tunnel: w278 -> [w403 _]
          tunnel: w279 -> [w398 _]
          frame False {
            n234 = call <userlib>:"LV_to_int_time.vi"("Time Stamp"=w403) -> ("Integer Time"=w397:i64)  [unwired: 8 in, 1 out]
            n235 = Bundle By Name(cluster=T5 {"Data"=[], "Integer Timestamp"=0, "Signal Length"=0, "DCS_ID"=0, "Role ID"=enum."First_Detector"} ("Cluster"), "Data"=w404, "Integer Timestamp"=w397, "Signal Length"=w398, "DCS_ID"=w397, "Role ID"=Role_ID."DCS 2") -> (w407:T5)
            n236 = Equal?(x="Tab Control", y=T1."Engineering Graphs") -> (x = y?=w399:bool)
            n237 = Build Array(w407) -> (w406:T7)
            n238 = case shown="True" w399 {
              tunnel: w409 -> [_ w414]
              tunnel: w404 -> [_ w413]
              frame False {
              }
              frame True {
                "Filtered Signals" <- w414
                "Unfiltered Signals" <- w413
              }
            }
            n239 = disable-structure shown="Disabled" {
              disable-tunnel: w406 -> [w412 _]
              disable-tunnel: "Waveform Path" -> [w411 _]
              disable-tunnel: w397 -> [w410 _]
              frame Disabled {
                n240 = call <userlib>:"DCS_write_signal_hdf5.vi"("Index"=w410, "Save Path"=w411, "Signal array"=w412) -> ()  [unwired: 8 in, 1 out]
              }
              frame Enabled {
              }
            }
          }
          frame True {
          }
        }
        n241 = Not A Number/Path/Refnum?(number/path/refnum=w365) -> (NaN/Path/Refnum?=w379:bool[])
        n242 = Or Array Elements(Boolean array=w379) -> (logical OR=w364:bool)
        n243 = case shown="False" w364 {
          tunnel: w380 -> [w958 w975]
          tunnel: [w953 w975] -> w309
          tunnel: w332 -> [w952 _]
          tunnel: w365 -> [w948 _]
          tunnel: w280 -> [w951 w974]
          tunnel: [w950 w974] -> w326
          tunnel: w358 -> [w949 w973]
          tunnel: [w947 w973] -> w335
          tunnel: w293 -> [w941 w972]
          tunnel: [w941 w972] -> w314
          tunnel: w284 -> [w942 _]
          tunnel: w278 -> [w939 _]
          frame False {
            n244 = Build Array (concatenate)(w949, w948) -> (w947:dbl[][])
            n245 = Index Array(array=w948, index=0) -> (element=w945:dbl)
            n246 = Index Array(array=w948, index=1) -> (element=w944:dbl)
            n247 = Search 1D Array(1D array=w952, element=w945) -> (index of element=w957:i32)  [unwired: 1 in]
            n248 = Search 1D Array(1D array=w952, element=w944) -> (index of element=w956:i32)  [unwired: 1 in]
            n249 = call <userlib>:"LV_to_int_time.vi"("Time Stamp"=w939) -> ("Integer Time"=w940:i64)  [unwired: 8 in, 1 out]
            n250 = disable-structure shown="Disabled" {
              disable-tunnel: [w966 _] -> w946
              disable-tunnel: w945 -> [w964 _]
              disable-tunnel: w944 -> [w963 _]
              disable-tunnel: w940 -> [w962 _]
              frame Disabled {
                # "DCS points DB stuff"
                n251 = Bundle By Name(cluster=T6 {"Integer Timestamp"=8, "X"=2.0, "Y"=3.0, "DCS spot ID"=0} ("DCS points"), "Integer Timestamp"=w962, "X"=w964, "Y"=w963) -> (w966:T6)
              }
              frame Enabled {
              }
            }
            n252 = Index Array(array=w958, index (row)=w957, index (col)=w956) -> (element=w955:dbl)
            n253 = Increment(x=w951) -> (x+1=w950:i32)
            n254 = Increment(x=w955) -> (x+1=w954:dbl)
            n255 = Replace Array Subset(array=w958, new element=w954, index (row)=w957, index (col)=w956) -> (w953:dbl[][])
            n256 = disable-structure shown="Disabled" {
              disable-tunnel: w946 -> [w961 _]
              frame Disabled {
                n257 = call <userlib>:"post_dcs_points.vi"("DCS points"=w961) -> ()  [unwired: 10 in, 1 out]
              }
              frame Enabled {
              }
            }
            n258 = case shown="True" "Record XY" {
              tunnel: w945 -> [_ w971]
              tunnel: w944 -> [_ w970]
              tunnel: "XY and Max" -> [_ w969]
              tunnel: w942 -> [_ w968]
              tunnel: w940 -> [_ w967]
              frame False {
              }
              frame True {
                n259 = call <userlib>:"Write_XY_Max.vi"("Numeric 2"=w971, "Numeric"=w970, "Integer Time"=w967, "X-Y position"=w968, "XY and Max"=w969) -> ()  [unwired: 7 in]
              }
            }
          }
          frame True {
          }
        }
        n260 = local read "Tab Control"() -> (w301:T1)
        n261 = Equal?(x=w301, y=T1."DCS") -> (x = y?=w299:bool)
        n262 = case shown="True" w299 {
          tunnel: w309 -> [_ w748]
          frame False {
          }
          frame True {
            n263 = Array Max & Min(array=w748) -> (max value=w747:dbl)  [unwired: 3 out]
            n264 = Index Array(array="Color bar Control") -> (element=w756:cluster{dbl, u32})  [unwired: 1 in]
            n265 = Bundle(cluster=w756, 0.0, u32 0) -> (w757:cluster{dbl, u32})
            n266 = Bundle(cluster=w756, w747, u32 16448250) -> (w754:cluster{dbl, u32})
            n267 = Bundle(cluster=w756, 1.0, u32 16860) -> (w755:cluster{dbl, u32})
            n268 = Build Array(w757, w755, w754) -> (w746:cluster{dbl, u32}[])
            n269 = local write "Color bar Control"(w746) -> ()
            n270 = property on="Intensity Graph" class="IntGraph (strict)"("ZScale.MarkerVals[]"="Color bar Control") -> ()  [unwired: 2 in, 2 out]
            "Intensity Graph" <- w748
          }
        }
        n271 = Equal To 0?(x=w326) -> (x = 0?=w362:bool)
        n272 = local read "Particle Limit"() -> (w330:i64)
        n273 = Select(t=-1, s=w362, f=w326) -> (s? t:f=w329:i32)
        n274 = Quotient & Remainder(x=w308, y=10) -> (x-y*floor(x/y)=w351:i32)  [unwired: 1 out]
        n275 = Equal To 0?(x=w351) -> (x = 0?=w306:bool)
        n276 = Quotient & Remainder(x=w329, y=w330) -> (x-y*floor(x/y)=w360:i64)  [unwired: 1 out]
        n277 = Quotient & Remainder(x=w329, y="# of shots to calculate spot") -> (x-y*floor(x/y)=w328:i32)  [unwired: 1 out]
        n278 = case shown="True" w306 {
          tunnel: w352 -> [w870 w877]
          tunnel: [w870 w874] -> w338
          tunnel: [w869 w873] -> w337
          tunnel: w339 -> [w869 w872]
          tunnel: w326 -> [_ w873]
          frame False {
          }
          frame True {
            n279 = Get Date/Time In Seconds() -> (seconds since 1Jan1904=w878:timestamp)
            n280 = To Double Precision Float(number=w878) -> (double precision float=w874:dbl)
            n281 = Subtract(x=w874, y=w877) -> (x-y=w876:dbl)
            n282 = Subtract(x=w873, y=w872) -> (x-y=w871:i32)
            n283 = Divide(x=w871, y=w876) -> (x/y=→"Avg. Freq. (Hz)":dbl)
          }
        }
        n284 = Equal To 0?(x=w328) -> (x = 0?=w321:bool)
        n285 = Subtract(x=w330, y=w360) -> (x-y=→"Countdown to\nnext track point":i64)
        n286 = Equal To 0?(x=w360) -> (x = 0?=w322:bool)
        n287 = event shown="[0] Timeout" {
          selector: _ -> [_ _ _]
          dyn-events: _ -> [_ _ _]
          timeout: 0 -> [_ _ _]
          tunnel: w332 -> [w810 w838 _]
          tunnel: w309 -> [w809 w839 _]
          tunnel: [w808 w837 w865] -> w341
          tunnel: w335 -> [w802 w829 _]
          tunnel: [w807 w836 dbl[][] []] -> w356
          tunnel: w326 -> [w800 w828 _]
          tunnel: [w800 w828 0] -> w325
          event Timeout {
            n288 = event-data() -> ()  [unwired: 1 in, 2 out]
            n289 = local read "Particle Limit"() -> (w803:i64)
            n290 = Array Size(array=w802) -> (size(s)=w806:i32[])
            n291 = Index Array(array=w806, index=0) -> (element=w804:i32)
            n292 = Greater?(x=w804, y=w803) -> (0:w801:bool)
            n293 = case shown="True" w801 {
              tunnel: w810 -> [_ w823]
              tunnel: w809 -> [w812 w818]
              tunnel: [w812 w817] -> w808
              tunnel: w802 -> [w811 w816]
              tunnel: [w811 w813] -> w807
              frame False {
              }
              frame True {
                n294 = Delete From Array(array=w816, index (row)=0) -> (deleted portion=w814:dbl[], array with subset deleted=w813:dbl[][])  [unwired: 2 in]
                n295 = Index Array(array=w814, index=0) -> (element=w824:dbl)
                n296 = Index Array(array=w814, index=1) -> (element=w825:dbl)
                n297 = Search 1D Array(1D array=w823, element=w824) -> (index of element=w819:i32)  [unwired: 1 in]
                n298 = Search 1D Array(1D array=w823, element=w825) -> (index of element=w820:i32)  [unwired: 1 in]
                n299 = Index Array(array=w818, index (row)=w819, index (col)=w820) -> (element=w822:dbl)
                n300 = Decrement(x=w822) -> (x-1=w821:dbl)
                n301 = Replace Array Subset(array=w818, new element=w821, index (row)=w819, index (col)=w820) -> (w817:dbl[][])
              }
            }
          }
          event "Particle Limit": Value Change {
            n302 = event-data() -> ()  [unwired: 1 in, 2 out]
            n303 = Array Size(array=w829) -> (size(s)=w835:i32[])
            n304 = Index Array(array=w835, index=0) -> (element=w833:i32)
            n305 = Greater?(x=w833, y="Particle Limit") -> (0:w830:bool)
            n306 = Subtract(x=w833, y="Particle Limit") -> (x-y=w831:i64)
            n307 = case shown="True" w830 {
              tunnel: w839 -> [w841 w845]
              tunnel: w829 -> [w840 w847]
              tunnel: w838 -> [_ w846]
              tunnel: [w840 w844] -> w836
              tunnel: [w841 w843] -> w837
              tunnel: w831 -> [_ w842]
              frame False {
              }
              frame True {
                n308 = for {
                  N: w842 -> [_]
                  tunnel: w846 -> [w852]
                  shift-right: [w848] -> w843
                  shift-left: w845 -> [w851]
                  shift-right: [w849] -> w844
                  shift-left: w847 -> [w853]
                  n309 = Delete From Array(array=w853, index (row)=0) -> (deleted portion=w850:dbl[], array with subset deleted=w849:dbl[][])  [unwired: 2 in]
                  n310 = Index Array(array=w850, index=0) -> (element=w859:dbl)
                  n311 = Index Array(array=w850, index=1) -> (element=w860:dbl)
                  n312 = Search 1D Array(1D array=w852, element=w859) -> (index of element=w855:i32)  [unwired: 1 in]
                  n313 = Search 1D Array(1D array=w852, element=w860) -> (index of element=w856:i32)  [unwired: 1 in]
                  n314 = Index Array(array=w851, index (row)=w855, index (col)=w856) -> (element=w858:dbl)
                  n315 = Decrement(x=w858) -> (x-1=w857:dbl)
                  n316 = Replace Array Subset(array=w851, new element=w857, index (row)=w855, index (col)=w856) -> (w848:dbl[][])
                }
              }
            }
          }
          event "Clear Spot/Track": Value Change {
            w866 = 49 ("dimension size")
            n317 = event-data() -> ()  [unwired: 1 in, 2 out]
            n318 = local write "Clear Spot/Track"(FALSE ("Clear Spot/Track")) -> ()
            n319 = Initialize Array(0.0 ("element"), w866, w866) -> (w865:dbl[][])
          }
        }
        n320 = case shown="True" "Save Spot Image" {
          tunnel: w281 -> [w785 w795]
          tunnel: [w785 w794] -> w282
          frame False {
          }
          frame True {
            n321 = Format Into String(format string="%03d", initial string="Image", w795) -> (resulting string=w791:string)  [unwired: 1 in, 1 out]
            n322 = Concatenate Strings(w791, ".png" ("string")) -> (w792:string)
            n323 = Build Path(base path="Spot Save Folder", name or relative path=w792) -> (appended path=w793:path)
            n324 = invoke on="Intensity Graph" class="IntGraph (strict)" method="Get Image"("image depth"=32 ("Image Depth")) -> ("image data"=w789:T8)  [unwired: 5 in, 5 out]
            n325 = call <vilib>:"Check if File or Folder Exists.vi"("path"="Spot Save Folder") -> ("file or folder exists?"=w786:bool)  [unwired: 8 in, 2 out]
            n326 = Increment(x=w795) -> (x+1=w794:i32)
            n327 = case shown="True" w786 {
              tunnel: w793 -> [_ w799]
              tunnel: w789 -> [_ w798]
              frame False {
              }
              frame True {
                n328 = call <vilib>:"Write PNG File.vi"("image data"=w798, "path to PNG file"=w799) -> ()  [unwired: 8 in, 2 out]
              }
            }
          }
        }
        n329 = for {
          tunnel: w341 -> [w932] mode=indexing
          tunnel: [w930] -> w378 mode=indexing
          tunnel: [w929] -> w377 mode=indexing
          i -> [w931]
          n330 = for {
            tunnel: w932 -> [w934] mode=indexing
            tunnel: w931 -> [w937]
            tunnel: [w935] -> w929 mode=indexing
            tunnel: [w933] -> w930 mode=indexing
            i -> [w936]
            n331 = Multiply(x=w934, y=w937) -> (x*y=w933:dbl)
            n332 = Multiply(x=w934, y=w936) -> (x*y=w935:dbl)
          }
        }
        n333 = Add Array Elements(numeric array=w341) -> (sum=w344:dbl)
        "# of Particles\nin Spot" <- w344
        n334 = Add Array Elements(numeric array=w378) -> (sum=w376:dbl)
        n335 = Add Array Elements(numeric array=w377) -> (sum=w375:dbl)
        n336 = Divide(x=w376, y=w344) -> (x/y=w374:dbl)
        n337 = Divide(x=w375, y=w344) -> (x/y=w373:dbl)
        n338 = Subtract(x=w374, y=24.0) -> (x-y=w367:dbl)
        n339 = Subtract(x=w373, y=24.0) -> (x-y=w371:dbl)
        n340 = Divide(x=w367, y=2.0) -> (x/y=w312:dbl)
        n341 = Divide(x=w371, y=2.0) -> (x/y=w311:dbl)
        n342 = property on="Intensity Graph" class="IntGraph (strict)"(error in=w314, "Active Cursor"=u32 0, "Cursor.Cursor X"=w312, "Cursor.Cursor Y"=w311) -> (error out=w313:errorcluster)  [unwired: 1 in, 1 out]
        n343 = Build Array(w312, w311) -> (w355:dbl[])
        "Current Spot Pos" <- w355
        n344 = disable-structure shown="Disabled" {
          disable-tunnel: w368 -> [w385 _]
          disable-tunnel: [w384 _] -> w340
          disable-tunnel: [w383 _] -> w336
          disable-tunnel: "Load old position\nto Orange Cursor" -> [w382 _]
          disable-tunnel: w293 -> [w381 _]
          frame Disabled {
            n345 = case shown="True" w382 {
              tunnel: [w387 w392] -> w384
              tunnel: w385 -> [w387 w389]
              tunnel: w381 -> [w386 w394]
              tunnel: [w386 w393] -> w383
              frame False {
              }
              frame True {
                # "DCS DB loading stuff"
                n346 = call <userlib>:"querey dcs spot.vi"("error in (no error)"=w394) -> ("Spot"=w388:T3, "Cancel loading"=w391:bool, "error out"=w393:errorcluster)  [unwired: 15 in, 1 out]
                n347 = Unbundle By Name(w388) -> ("Spot X"=w396:dbl, "Spot Y"=w395:dbl)
                n348 = Build Array(w396, w395) -> (w390:dbl[])
                n349 = Select(t=w389, s=w391, f=w390) -> (s? t:f=w392:dbl[])
              }
            }
          }
          frame Enabled {
          }
        }
        n350 = case shown="False" w321 {
          tunnel: w357 -> [w881 w915]
          tunnel: [w881 w883] -> w354
          tunnel: w309 -> [_ w896]
          tunnel: w345 -> [w880 w895]
          tunnel: w355 -> [_ w893]
          tunnel: [w880 w894] -> w353
          tunnel: w344 -> [_ w887]
          tunnel: [w879 w886] -> w343
          tunnel: w314 -> [w879 w884]
          tunnel: w322 -> [_ w882]
          frame False {
          }
          frame True {
            w906 = sgl 0.0 ("element")
            w907 = sgl 2.0 ("element")
            # "DCS Spots DB stuff"
            n351 = Build Array (concatenate)(w895, w893) -> (w894:dbl[][])
            n352 = Array Max & Min(array=w896) -> (max value=w909:dbl, max index (indices)=w908:i32[])  [unwired: 2 out]
            n353 = Array Size(array=w896) -> (size(s)=w912:i32[])
            n354 = Index Array(array=w893) -> (element #1=w892:dbl, element #2=w891:dbl)  [unwired: 2 in]
            n355 = Multiply Array Elements(1:w912) -> (0:w913:i32)
            n356 = To Variant(anything=w912) -> (Variant=w911:variant)
            n357 = Build Array (concatenate)(w909, w908, w907, w907, w906, w906) -> (w905:dbl[])
            n358 = Reshape Array(w896, w913) -> (w910:dbl[])
            n359 = vi-ref <userlib>:"2DGaussianRotationModelwithOffset.vi"() -> (w914:refnum<vi>)
            n360 = call-poly <vilib>:"Nonlinear Curve Fit.vi"("Y"=w910, "f(x,a)"=w914, "data"=w911, "initial parameters"=w905, "error in (no error)"=w884, "termination"=cluster{"max iteration":i32, "tolerance":dbl} {"max iteration"=1000, "tolerance"=1e-08}) -> ("best fit parameters"=w898:dbl[], "error out"=w885:errorcluster)  [unwired: 4 in, 4 out]
            n361 = Array Subset(array=w898, index=3, length=2) -> (w901:dbl[])
            n362 = Divide(x=24.0 ("y"), y=49.0) -> (x/y=w897:dbl)
            n363 = Multiply(x=w901, y=w897) -> (x*y=w890:dbl[])
            "Spot Widths" <- w890
            n364 = Build Array (concatenate)(w915, w890) -> (w883:dbl[][])
            n365 = Index Array(array=w890) -> (element #1=w889:dbl, element #2=w888:dbl)  [unwired: 2 in]
            n366 = case shown="True" w882 {
              tunnel: w892 -> [_ w924]
              tunnel: w891 -> [_ w923]
              tunnel: w889 -> [_ w922]
              tunnel: w888 -> [_ w921]
              tunnel: w887 -> [_ w920]
              tunnel: [w916 w918] -> w886
              tunnel: w885 -> [w916 w917]
              frame False {
              }
              frame True {
                n367 = Get Date/Time In Seconds() -> (seconds since 1Jan1904=w925:timestamp)
                n368 = call <userlib>:"LV_to_int_time.vi"("error in (no error)"=w917, "Time Stamp"=w925) -> ("error out"=w919:errorcluster, "Integer Time"=w928:i64)  [unwired: 7 in]
                n369 = Bundle By Name(cluster=T3 {"DCS spot ID"=0, "Integer Timestamp"=2, "Spot X"=3.0, "Spot Y"=4.0, "Spot Width X"=0.0, "Spot Width Y"=0.0, "Spot Size"=0, "Experiment Settings ID"=0} ("dcs_spot"), "Integer Timestamp"=w928, "Spot X"=w924, "Spot Y"=w923, "Spot Width X"=w922, "Spot Width Y"=w921, "Spot Size"=w920) -> (w927:T3)
                n370 = call <userlib>:"post_dcs_spot.vi"("error in (no error)"=w919, "dcs_spot"=w927) -> ("error out"=w918:errorcluster)  [unwired: 9 in]
              }
            }
          }
        }
        n371 = Subtract(x="Orange Cursor Position", y=w355) -> (x-y=w350:dbl[])
        n372 = Select(t=w340, s="Load old position\nto Orange Cursor", f=w355) -> (s? t:f=w318:dbl[])
        n373 = Multiply(x=w350, y=8.6106) -> (x*y=w348:dbl[])
        n374 = Or(x="Load old position\nto Orange Cursor", y="Set Orange Cursor\nto current position") -> (x .or. y?=w317:bool)
        n375 = case shown="True" w317 {
          tunnel: "Orange Cursor Position" -> [w777 _]
          tunnel: w318 -> [_ w784]
          tunnel: 1 -> [w774 w782]
          tunnel: w313 -> [w773 w779]
          tunnel: [w772 w778] -> w315
          frame False {
            n376 = Index Array(array=w777) -> (element #1=w776:dbl, element #2=w775:dbl)  [unwired: 2 in]
            n377 = property on="Intensity Graph" class="IntGraph (strict)"(error in=w773, "Active Cursor"=w774, "Cursor.Cursor X"=w776, "Cursor.Cursor Y"=w775) -> (error out=w772:errorcluster)  [unwired: 1 in, 1 out]
          }
          frame True {
            n378 = Index Array(array=w784) -> (element #1=w781:dbl, element #2=w780:dbl)  [unwired: 2 in]
            n379 = local write "Set Orange Cursor\nto current position"(FALSE ("Set Orange Cursor\nto current position")) -> ()
            n380 = local write "Orange Cursor Position"(w784) -> ()
            n381 = property on="Intensity Graph" class="IntGraph (strict)"(error in=w779, "Active Cursor"=w782, "Cursor.Cursor X"=w781, "Cursor.Cursor Y"=w780) -> (error out=w778:errorcluster)  [unwired: 1 in, 1 out]
          }
        }
        n382 = Divide(x=w348, y=2.0) -> (x/y=→"Laser spot\nMove (mm)":dbl[])
        n383 = local read "Tab Control"() -> (w303:T1)
        n384 = local read "Tab Control"() -> (w320:T1)
        n385 = Equal?(x=w303, y=T1."DCS") -> (x = y?=w302:bool)
        n386 = Equal?(x=w320, y=T1."Spot Size Tracking") -> (x = y?=w305:bool)
        n387 = case shown="True" w302 {
          tunnel: w353 -> [_ w769]
          tunnel: w343 -> [w759 w768]
          tunnel: [w759 w767] -> w342
          frame False {
          }
          frame True {
            n388 = Index Array(array=w769, index (col)=0 ("disabled index (col)")) -> (element=w763:dbl[])  [unwired: 1 in]
            n389 = Index Array(array=w769, index (col)=1 ("disabled index (col)")) -> (element=w761:dbl[])  [unwired: 1 in]
            n390 = call "Convert to Dynamic Data"("Array"=w763) -> ("Dynamic Data Type"=w762:dynamicdata)  [unwired: 3 in]
            n391 = call "Convert to Dynamic Data2"("Array"=w761) -> ("Dynamic Data Type"=w760:dynamicdata)  [unwired: 3 in]
            n392 = call "Build XY Graph"("error in (no error)"=w768, "Y Input"=w760, "X Input"=w762) -> ("error out"=w767:errorcluster, "XY Graph"=→"XY Graph":cluster{"Y":dbl[], "Y":dbl[]}[])  [unwired: 2 in, 5 out]
          }
        }
        n393 = case shown="True" w305 {
          tunnel: w354 -> [_ w771]
          frame False {
          }
          frame True {
            n394 = Transpose 2D Array(2D array=w771) -> (transposed array=→"Spot Size over time":dbl[][])
          }
        }
        n395 = Merge Errors(w342, w315, w336) -> (w331:errorcluster)
        "Running Errors" <- w293
      }
      n396 = Not(x=w47) -> (.not. x?=w41:bool)
      n397 = Not Equal To 0?(x=w42) -> (x != 0?=w39:bool)
      n398 = And(x=w39, y=w41) -> (x .and. y?=w40:bool)
      n399 = case shown="True" w40 {
        tunnel: w55 -> [_ w246]
        tunnel: w46 -> [_ w242]
        frame False {
        }
        frame True {
          n400 = Index Array(array=w246) -> (element #1=w245:dbl, element #2=w244:dbl)  [unwired: 2 in]
          n401 = Array Size(array=w242) -> (size(s)=w243:i32[])
          n402 = Get Date/Time In Seconds() -> (seconds since 1Jan1904=w248:timestamp)
          n403 = Index Array(array=w243) -> (element=w241:i32)  [unwired: 1 in]
          n404 = call <userlib>:"LV_to_int_time.vi"("Time Stamp"=w248) -> ("Integer Time"=w247:i64)  [unwired: 8 in, 1 out]
          n405 = disable-structure shown="Disabled" {
            disable-tunnel: w247 -> [w260 _]
            disable-tunnel: w245 -> [w257 _]
            disable-tunnel: w244 -> [w256 _]
            disable-tunnel: w242 -> [w255 _]
            disable-tunnel: w241 -> [w254 _]
            disable-tunnel: 0 ("disabled index (col)") -> [w252 _]
            disable-tunnel: 1 ("disabled index (col)") -> [w251 _]
            frame Disabled {
              # "Stuff to post last spot on shutdown"
              n406 = local read "# of Particles\nin Spot"() -> (w249:dbl)
              n407 = Index Array(array=w255, index (row) #1=w254, index (col) #1=w252, index (row) #2=w254, index (col) #2=w251) -> (element #1=w253:dbl, element #2=w250:dbl)
              n408 = Bundle By Name(cluster=T3 {"DCS spot ID"=0, "Integer Timestamp"=2, "Spot X"=3.0, "Spot Y"=4.0, "Spot Width X"=0.0, "Spot Width Y"=0.0, "Spot Size"=0, "Experiment Settings ID"=0} ("dcs_spot"), "Integer Timestamp"=w260, "Spot X"=w257, "Spot Y"=w256, "Spot Width X"=w253, "Spot Width Y"=w250, "Spot Size"=w249) -> (w258:T3)
              n409 = call <userlib>:"post_dcs_spot.vi"("dcs_spot"=w258) -> ()  [unwired: 10 in, 1 out]
            }
            frame Enabled {
            }
          }
        }
      }
    }
    frame Error {
    }
  }
  "error out" <- w13
